vi "Protocol Read.vi"(8 "error in":errorcluster, 9 "timeout":i32=10000, 10 "bytes to read":i32, 11 "protocol layer in":refnum<class "Serial Slave.lvclass">) -> (0 "error out":errorcluster, 1 "timed out?":bool, 2 "data":u8[](array[numeric]), 3 "protocol layer out":refnum<class "Serial Slave.lvclass">)   [LabVIEW 2012, in "Serial Slave.lvclass"]
doc: "This provides an interface for reading from a network bus."
uses:
  Serial Slave.lvclass
  Serial Slave.lvclass/Serial Slave.ctl
  Serial Shared Components/Serial Shared Components.lvlib
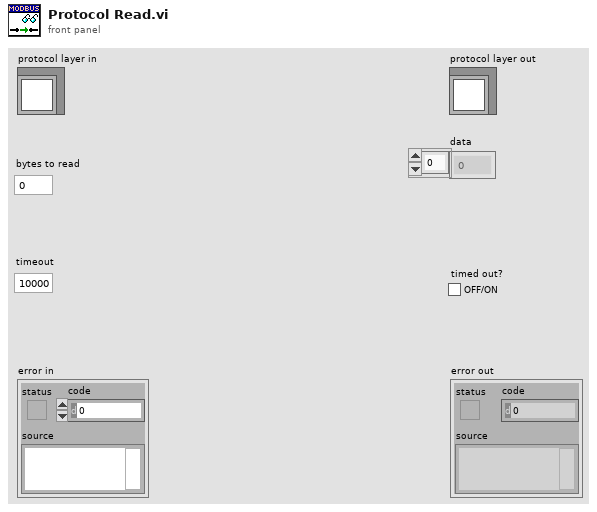
[diagram p1: front panel]
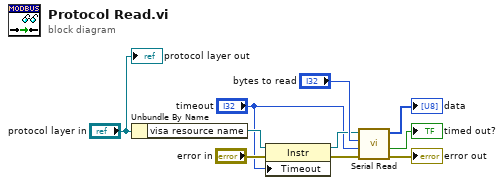
[diagram p0: block diagram]
diagram:
  n1 = Unbundle By Name("protocol layer in") -> ("visa resource name"=w3:refnum<visa-resource-name>)
  n2 = property class="Instr"(reference=w3, error in="error in", "Timeout"="timeout") -> (reference out=w2:refnum<visa-resource-name>, error out=w4:errorcluster)
  n3 = call "Serial Read.vi"("error in"=w4, "timeout (ms)"="timeout", "bytes to read"="bytes to read", "Visa Resource"=w2) -> ("error out"=→"error out":errorcluster, "timed out?"=→"timed out?":bool, "data"=→"data":u8[])  [unwired: 5 in]
  "protocol layer out" <- "protocol layer in"
